vi "v2.vi"() -> ()   [LabVIEW 2012]
panel:
  out "data":dbl
  in  "stop (F)":bool
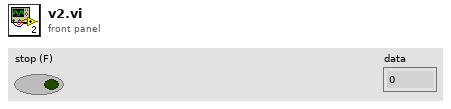
[diagram p1: front panel]
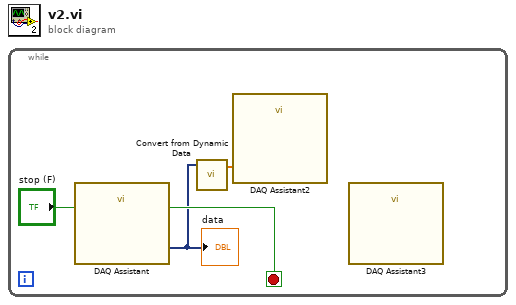
[diagram p0: block diagram]
diagram:
  n1 = while {
    stop <- w3 stop-if-true
    n2 = call "DAQ Assistant"("stop (F)"="stop (F)") -> ("data"=w2:dynamicdata, "stopped"=w3:bool)  [unwired: 15 in, 2 out]
    "data" <- w2
    n3 = call "Convert from Dynamic Data"("Dynamic Data Type"=w2) -> ("Array"=w1:dbl[])  [unwired: 3 in]
    n4 = call "DAQ Assistant2"("data"=w1) -> ()  [unwired: 17 in, 2 out]
    n5 = call "DAQ Assistant3"() -> ()  [unwired: 17 in, 3 out]
  }
